vi "muCTA.vi"() -> (0 "DAQ Error":errorcluster)   [LabVIEW 2018]
uses:
  Globals/Meas_global.vi
panel:
  out "Waveform Graph":dbl[][](graph)
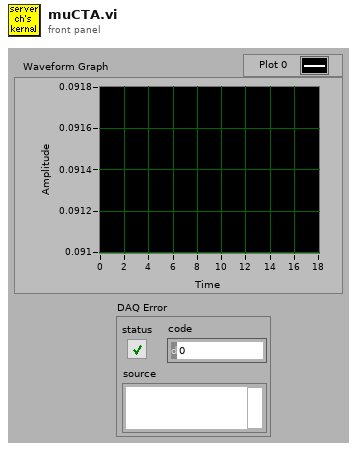
[diagram p1: front panel]
types:
  T1 = typedef "Setup.ctl" = enum16{"Run Program", "Show Setup", "Save Current Setup", "Setup Front Panel"}
  T2 = typedef "Analysis_info_cluster.ctl" = cluster{"Colour":u32, "Inst type":T3, "Inst name":string, "Symbol":string, "Code name":string, "Extra Info":string, "Inst Array":T4, "Extra Titles":string[], "Extra Values":string[], "U":dbl, "u^2":dbl, "u^3":dbl, "u^4":dbl, "Skew_u":dbl, "Kurt_u":dbl, "Sd Error in Mean":dbl, "% u'/U":dbl, "X":dbl, "Y":dbl, "Z":dbl, "Timescale integral Estimate":dbl, "Sd Error in Variance":dbl, "Calib File":path, "Calib Constants":dbl[], "Output Position":bool, "Stats":enum16{"None", "Basic", "Full"}, "Av Sampling Rate":dbl, "Av No of Samples":dbl, "Total Meas Time (s)":dbl, "ADAM Ch Name":string, "Max value":dbl, "Min value":dbl, "Req Sample Rate Hz":dbl, "Sync Delay Time (s)":dbl, "Ch No":i16, "Device":string, "Use Latest Calib":bool, "Port":string, "Metadata Ch Names":string[], "Metadata Ch Values":string[]}
  T3 = typedef "Inst_type.ctl" = enum16{"Propeller anemometer", "Raw voltage", "Pressure Transducer", "Pitot-static tube", "Preston tube", "Hot wire", "Cross wire 1", "Cross wire 2", "Generic Linear", "Generic Polynomial", "Generic BackPoly", "Fast FID", "Thermocouple", "Cold wire", "Pulsed Wire", "LDA Vel", "LDA Tran time", "LDA Arr time", "Microphone"}
  T4 = typedef "Instrument_Array.ctl" = enum16{"PWA", "LDA", "Analogue"}
  T5 = typedef "Rendezvous RefNum" = refnum<k1>
  T6 = typedef "Device ID port info.ctl" = cluster{"Ch No":i16[], "Req Sampling Rate":dbl[], "Port":string, "Index":i32[]}
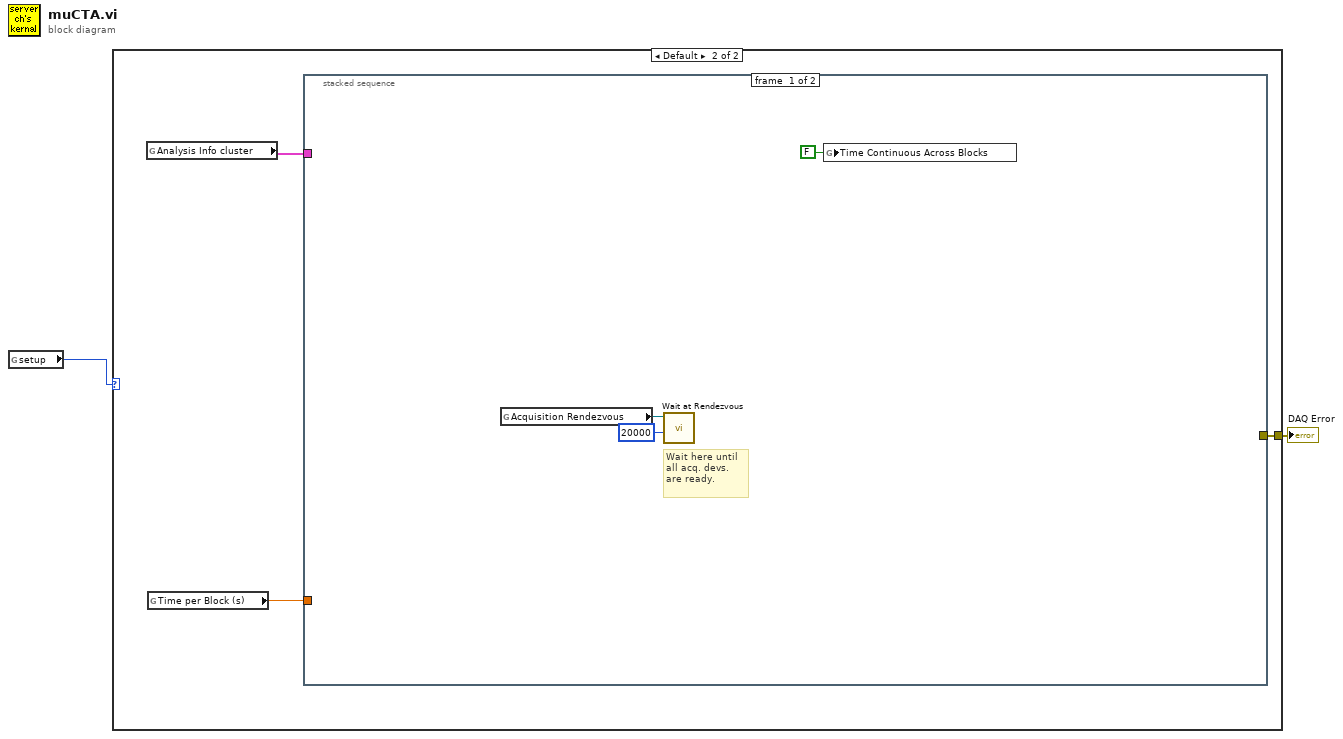
[diagram p0: block diagram]
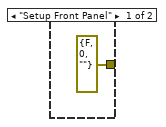
[diagram p2: hidden frame]
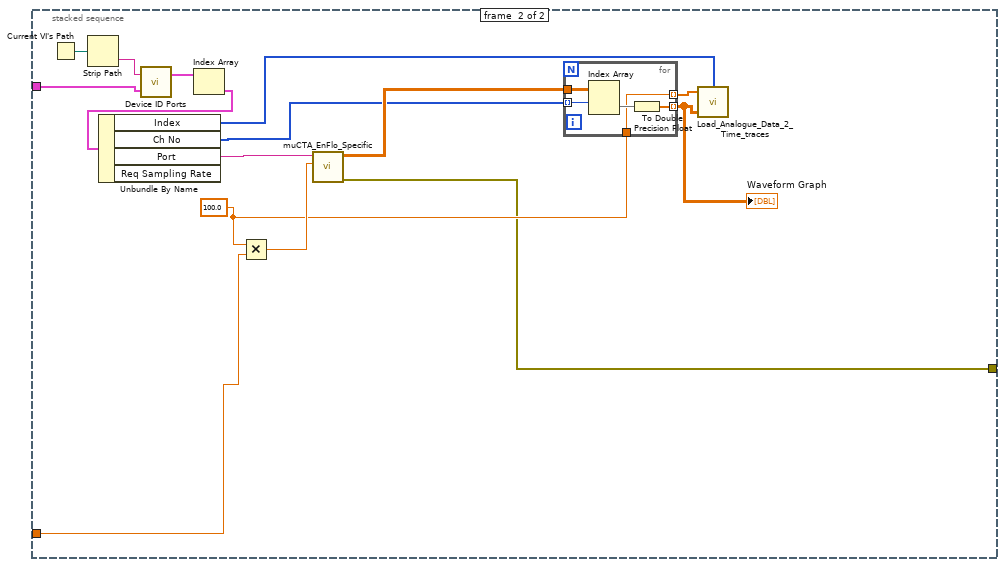
[diagram p3: hidden frame]
diagram:
  n1 = global read "Meas_global.vi" "setup"() -> (w1:T1)
  n2 = case shown="Default" w1 {
    tunnel: [errorcluster {"status"=FALSE, "code"=0, "source"=""} ("DAQ Error") w5] -> w2
    frame "Setup Front Panel" {
    }
    frame Default {
      n3 = global read "Meas_global.vi" "Analysis Info cluster"() -> (w6:T2[])
      n4 = global read "Meas_global.vi" "Time per Block (s)"() -> (w4:dbl)
      n5 = stacked-sequence {
        tunnel: w6 -> [_ w22]
        tunnel: [_ w11] -> w5
        tunnel: w4 -> [_ w18]
        frame #0 {
          # "Wait here until all acq. devs. are ready."
          n6 = global read "Meas_global.vi" "Acquisition Rendezvous"() -> (w8:T5)
          n7 = call <vilib>:"Wait at Rendezvous.vi"("ms timeout (-1)"=20000, "rendezvous"=w8) -> ()  [unwired: 3 in, 3 out]
          n8 = global write "Meas_global.vi" "Time Continuous Across Blocks"(FALSE ("Time Continuous across Blocks")) -> ()
        }
        frame #1 {
          w12 = 100.0 ("x")
          n9 = Current VI's Path() -> (path=w24:path)
          n10 = Strip Path(path=w24) -> (name=w23:string)  [unwired: 1 out]
          n11 = call "Device ID Ports.vi"("Analysis Info cluster"=w22, "Device ID"=w23) -> ("Device port info"=w21:T6[])  [unwired: 1 out]
          n12 = Index Array(array=w21) -> (element=w20:T6)  [unwired: 1 in]
          n13 = Unbundle By Name(w20) -> ("Index"=w13:i32[], "Ch No"=w14:i16[], "Port"=w19:string)  [unwired: 1 out]
          n14 = Multiply(x=w12, y=w18) -> (x*y=w17:dbl)
          n15 = call "muCTA_EnFlo_Specific.vi"("N samples"=w17, "VISA resource name"=w19) -> ("I/O error"=w11:errorcluster, "Data out"=w15:sgl[][])  [unwired: 3 in, 1 out]
          n16 = for {
            tunnel: w14 -> [w28] mode=indexing
            tunnel: w15 -> [w29]
            tunnel: w12 -> [w25]
            tunnel: [w26] -> w10 mode=indexing
            tunnel: [w25] -> w16 mode=indexing
            n17 = Index Array(array=w29, index (row)=w28) -> (element=w27:sgl[])  [unwired: 1 in]
            n18 = To Double Precision Float(number=w27) -> (double precision float=w26:dbl[])
          }
          "Waveform Graph" <- w10
          n19 = call "Load_Analogue_Data_2_Time_traces.vi"("Index"=w13, "Voltage Array"=w10, "Sampling Rate (Hz)"=w16) -> ()  [unwired: 3 in]
        }
      }
    }
  }
  "DAQ Error" <- w2
